vi "PicturePuzzleFinal.vi"() -> ()   [LabVIEW 2014]
panel:
  in  "Difficulty":i32(slide) scale=1.0..3.0
  in  "End Game":bool
  out "Game Array":picture[][](array[picture])
  # "Picture Puzzle!"
  # "Choose a level of difficulty and run the VI. Select to an image you want to turn into a puzzle and try not to\nget too frustrated!"
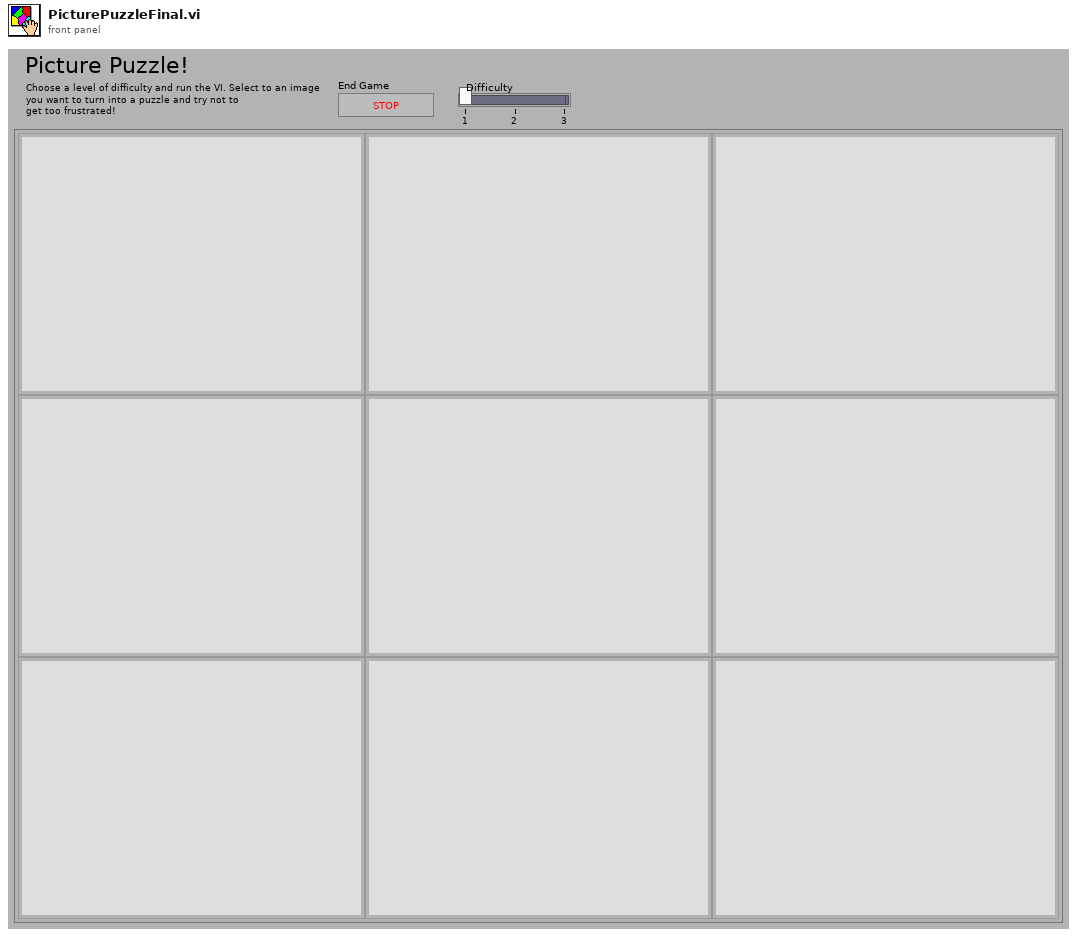
[diagram p1: front panel]
types:
  T1 = typedef "imagedata.ctl" = cluster{"image type":i32, "image depth":i32, "image":u8[], "mask":u8[], "colors":u32[], "Rectangle":cluster{"left":i16, "top":i16, "right":i16, "bottom":i16}}
  T2 = cluster{"Draw Image Size Y":i32, "Draw Image Size X":i32}
  T3 = cluster{"Numeric Control":i32, "Numeric Control":i32}
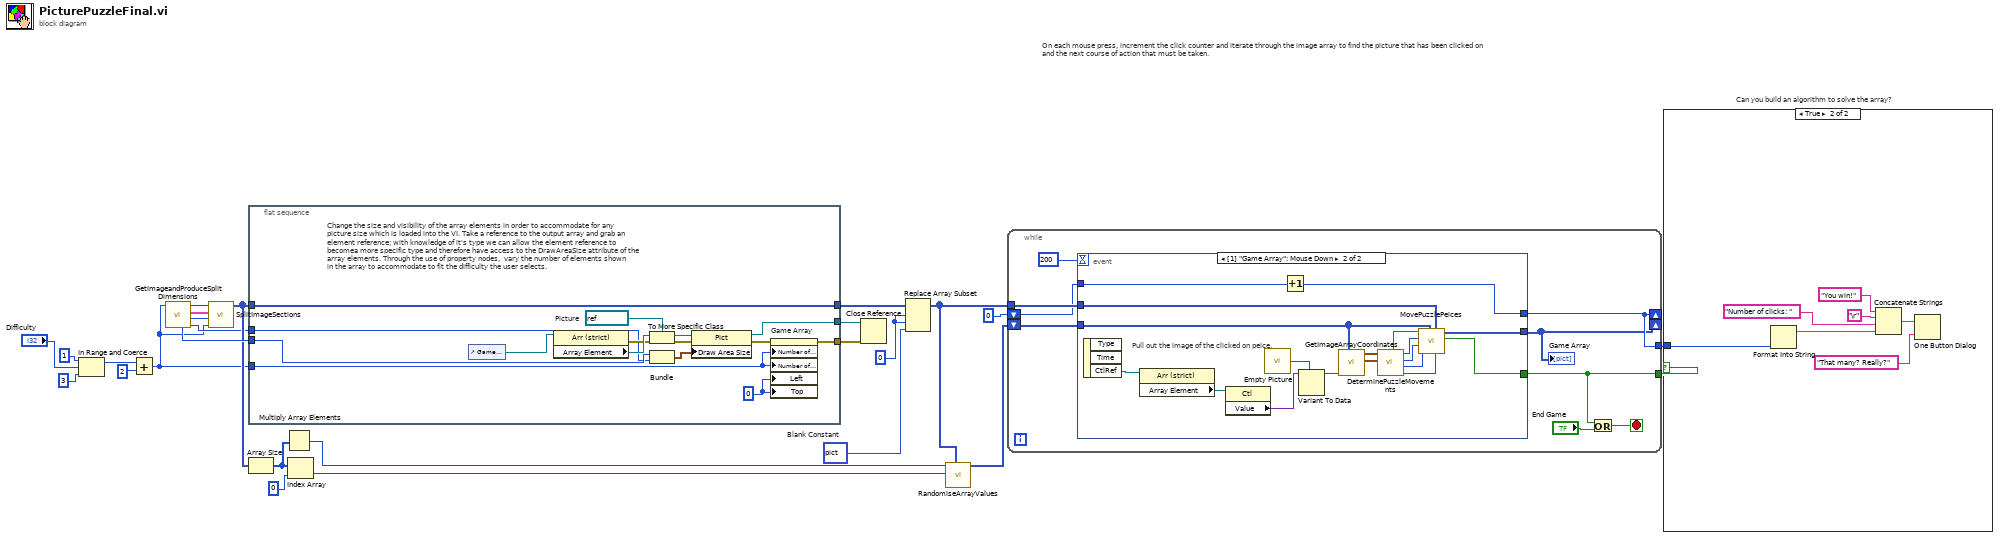
[diagram p0: block diagram]
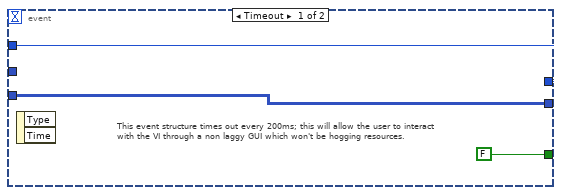
[diagram p3: hidden frame]
diagram:
  w15 = 0 ("index (row)")
  w16 = picture data[5B]  # Blank Constant
  # "Can you build an algorithm to solve the array?"
  # "On each mouse press, increment the click counter and iterate through the image array to find the picture that has been clicked on\nand the next course of action that must be taken."
  n1 = In Range and Coerce(upper limit=1, x="Difficulty", lower limit=3) -> (coerced(x)=w7:i32)  [unwired: 1 out]
  n2 = Add(x=w7, y=2) -> (x+y=w2:i32)
  n3 = call "GetImageandProduceSplitDimensions.vi"("Row/Column [].Length"=w2) -> ("Draw Image Size X"=w4:i32, "Image Subset Y Length"=w25:i32, "Selected Image"=w26:T1, "Image Subset X Length"=w24:i32, "Draw Image Size Y"=w20:i32)  [unwired: 6 in]
  n4 = call "SplitImageSections.vi"("Array Lenght (1D)"=w2, "Y Length"=w25, "Selected Image"=w26, "X Length"=w24) -> ("Chopped Image Array"=w8:picture[][])  [unwired: 7 in]
  n5 = flat-sequence {
    tunnel: w8 -> [w35]
    tunnel: [w35] -> w17
    tunnel: w20 -> [w34]
    tunnel: w4 -> [w28]
    tunnel: [w31] -> w18
    tunnel: [w33] -> w19
    tunnel: w2 -> [w30]
    frame #0 {
      w29 = 0 ("Position:Left")
      w38 = refnum<vi> refnum  # Picture
      # "Change the size and visibility of the array elements in order to accommodate for any \npicture size which is loaded into the VI. Take a reference to the output array and grab an \nelement reference; with knowledge of it's type we can allow the element reference to \nbecomea more specific type and therefore have access to the DrawAreaSize attribute of the\narray elements. Through the use of property nodes,  vary the number of elements shown\nin the array to accommodate to fit the difficulty the user selects."
      n6 = control-ref of="Game Array"() -> (w41:refnum<vi>)
      n7 = property class="Arr (strict)"(reference=w41) -> (error out=w39:errorcluster, "Array Element"=w40:refnum<vi>)  [unwired: 1 in, 1 out]
      n8 = To More Specific Class(target class=w38, reference=w40, error in=w39) -> (specific class reference=w37:refnum<vi>, error out=w36:errorcluster)
      n9 = Bundle("Draw Image Size Y"=w34, "Draw Image Size X"=w28) -> (w27:T2)  [unwired: 1 in]
      n10 = property class="Pict"(reference=w37, error in=w36, "Draw Area Size"=w27) -> (reference out=w33:refnum<vi>, error out=w32:errorcluster)
      n11 = property on="Game Array" class="Arr (strict)"(error in=w32, "Number of Columns"=w30, "Number of Rows"=w30, "Left"=w29, "Top"=w29) -> (error out=w31:errorcluster)  [unwired: 1 in, 1 out]
    }
  }
  n12 = Array Size(array=w8) -> (size(s)=w22:i32[])
  n13 = Multiply Array Elements(1:w22) -> (0:w21:i32)
  n14 = Index Array(array=w22, index=0) -> (element=w10:i32)
  n15 = Close Reference(reference=w19, error in (no error)=w18) -> ()  [unwired: 1 out]
  n16 = Replace Array Subset(array=w17, new element=w16, index (row)=w15, index (col)=w15) -> (w3:picture[][])
  n17 = call "RandomiseArrayValues.vi"("Original Image"=w3, "Maximum Array Width/Height"=w10, "Total Array Elements"=w21) -> ("Randomised Array"=w14:picture[][])  [unwired: 8 in]
  n18 = while {
    shift-right: [w42] -> _
    shift-left: w14 -> [w49]
    tunnel: w3 -> [w48]
    tunnel: [w43] -> w1
    tunnel: [w45] -> w13
    shift-right: [w45] -> _
    shift-left: 0 -> [w46]
    stop <- w47 stop-if-true
    n19 = event shown="[1] \"Game Array\": Mouse Down" {
      selector: _ -> [_ _]
      dyn-events: _ -> [_ _]
      timeout: 200 -> [_ _]
      tunnel: w49 -> [w53 w58]
      tunnel: [w53 w64] -> w42
      tunnel: w48 -> [_ w59]
      tunnel: [FALSE w63] -> w43
      tunnel: w46 -> [w51 w62]
      tunnel: [w51 w61] -> w45
      event Timeout {
        # "This event structure times out every 200ms; this will allow the user to interact\nwith the VI through a non laggy GUI which won't be hogging resources."
        n20 = event-data() -> ()  [unwired: 1 in, 2 out]
      }
      event "Game Array": Mouse Down {
        # "Pull out the image of the clicked on peice."
        n21 = event-data() -> ("CtlRef"=w71:refnum<vi>)  [unwired: 1 in, 2 out]
        n22 = property class="Arr (strict)"(reference=w71) -> ("Array Element"=w70:refnum<vi>)  [unwired: 1 in, 2 out]
        n23 = property class="Ctl"(reference=w70) -> ("Value"=w69:variant)  [unwired: 1 in, 2 out]
        n24 = call "Empty Picture"() -> ("empty picture"=w68:picture)
        n25 = Increment(x=w62) -> (x+1=w61:i32)
        n26 = Variant To Data(type=w68, Variant=w69) -> (data=w60:picture)  [unwired: 1 in, 1 out]
        n27 = call "GetImageArrayCoordinates.vi"("Current Puzzle Array"=w58, "Image Selected"=w60) -> ("White Location out"=w66:T3, "Peice Location out"=w67:T3)  [unwired: 8 in]
        n28 = call "DeterminePuzzleMovements.vi"("White Location In"=w66, "Peice Location In"=w67) -> ("Upper White Row Position"=w55:i32, "Current Peice Column"=w54:i32, "Current Peice Row"=w65:i32, "Lower White Column Position"=w56:i32, "Allow Peice Movement"=w57:bool)  [unwired: 5 in]
        n29 = call "MovePuzzlePeices.vi"("Upper White Row Position"=w55, "Solved Puzzle"=w59, "Current Puzzle State"=w58, "Current Selected Peice Column"=w54, "Current Selected Peice Row"=w65, "Lower White Coordinate"=w56, "Allow Peice Movement"=w57) -> ("Puzzle Finished"=w63:bool, "Updated Image Array"=w64:picture[][])  [unwired: 3 in]
      }
    }
    "Game Array" <- w42
    n30 = Or(x=w43, y="End Game") -> (x .or. y?=w47:bool)
  }
  n31 = case shown="True" w1 {
    tunnel: w13 -> [_ w76]
    frame False {
    }
    frame True {
      n32 = Format Into String(w76) -> (resulting string=w75:string)  [unwired: 3 in, 1 out]
      n33 = Concatenate Strings("You win!" ("message"), "\r", "Number of clicks: " ("string"), w75) -> (w77:string)
      n34 = One Button Dialog(message=w77, button name ("OK")="That many? Really?") -> ()  [unwired: 1 out]
    }
  }
